vi "GEOM_SortROILevels.vi"(6 "type":enum16{"any", "normal", "rotated"}(ring), 8 "index":i32, 9 "amplifiers":T1[](array[typedef]) {"fliped" items=["none", "horizontal", "vertical"]; "type" items=["LL", "LR", "UL", "UR"]}, 10 "how":enum16{"rows (y)", "columns (x)"}(ring)) -> (1 "totpix":u32, 2 "levels":cluster{"amplifiers":i32, "coord":i32}[](array[cluster]), 4 "totdata":i32)   [LabVIEW 2016]
uses:
  GEOM_Amplifier.ctl
  GEOM_AmpType.ctl
  GEOM_ROI.ctl
  GEOM_Coords.ctl
panel:
  out "sorted amplifiers":T1[](array[typedef]) {"fliped" items=["none", "horizontal", "vertical"]; "type" items=["LL", "LR", "UL", "UR"]}
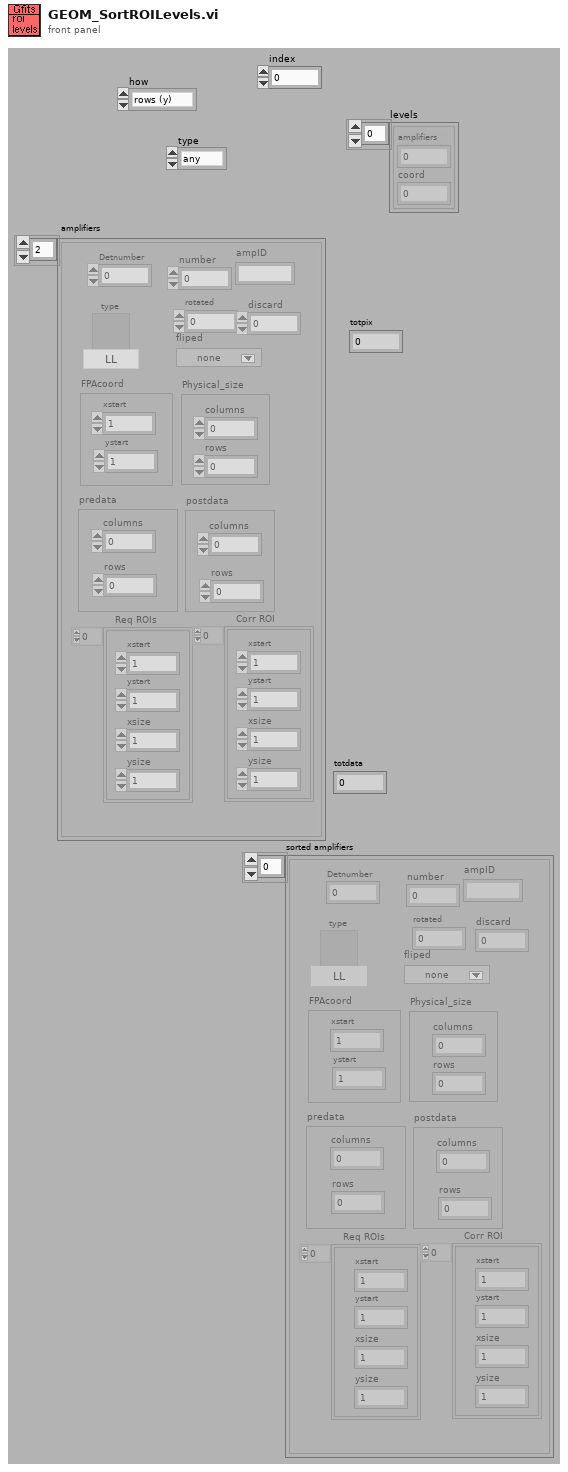
[diagram p1: front panel]
types:
  T1 = typedef "GEOM_Amplifier.ctl" = cluster{"number":i32, "type":T2, "rotated":i16, "fliped":u16, "FPAcoord":cluster{"xstart":i32, "ystart":i32}, "Physical_size":cluster{"columns":i32, "rows":i32}, "predata":cluster{"columns":i32, "rows":i32}, "postdata":cluster{"columns":i32, "rows":i32}, "Req ROIs":T3, "Corr ROI":T3, "Detnumber":i32, "ampID":string, "discard":i32}
  T2 = typedef "GEOM_AmpType.ctl" = u16
  T3 = typedef "GEOM_ROI.ctl" = T4[]
  T4 = typedef "GEOM_Coords.ctl" = cluster{"xstart":u32, "ystart":u32, "xsize":u32, "ysize":u32}
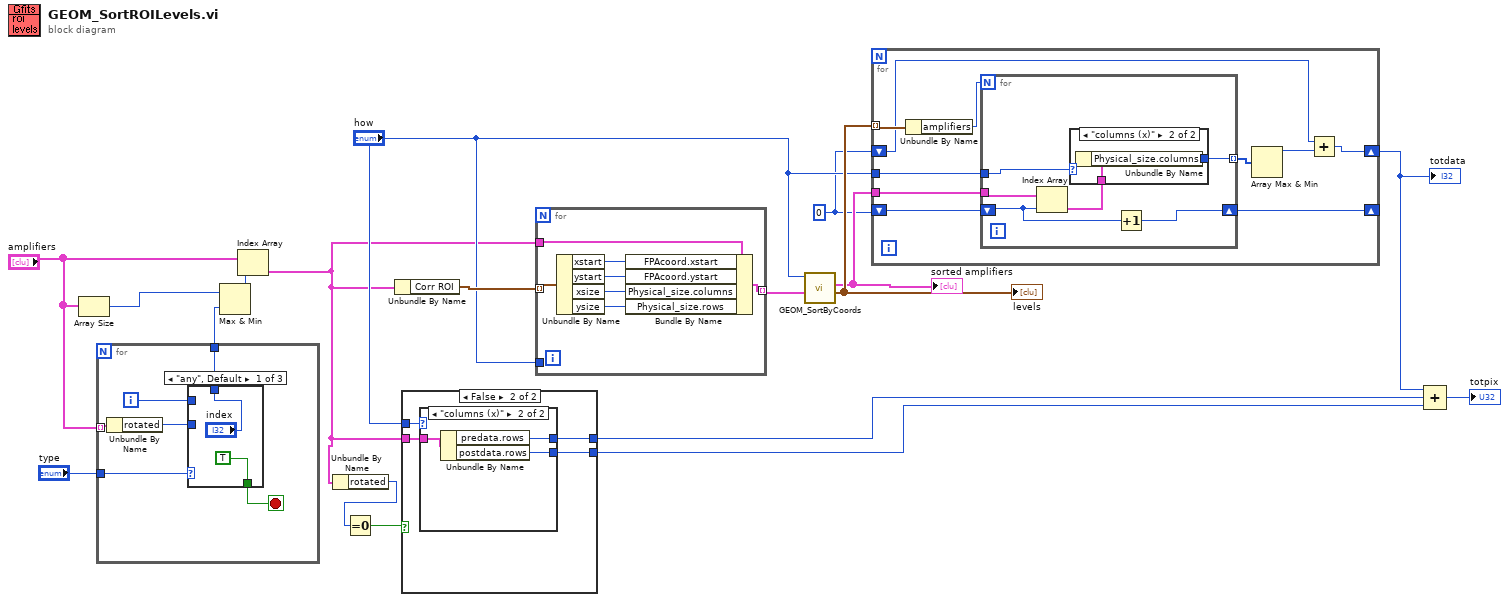
[diagram p0: block diagram]
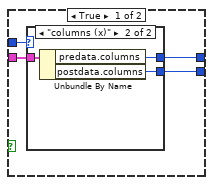
[diagram p2: hidden frame]
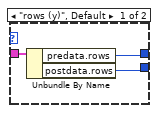
[diagram p3: hidden frame]
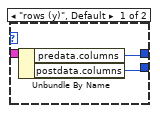
[diagram p4: hidden frame]
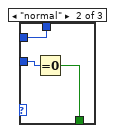
[diagram p5: hidden frame]
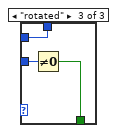
[diagram p6: hidden frame]
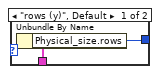
[diagram p7: hidden frame]
diagram:
  w11 = 0
  n1 = Array Size(array="amplifiers") -> (size(s)=w7:i32)
  n2 = for {
    tunnel: "amplifiers" -> [w24] mode=indexing
    tunnel: "type" -> [w23]
    tunnel: [w21] -> w5
    i -> [w20]
    stop <- w22 stop-if-true
    n3 = Unbundle By Name(w24) -> ("rotated"=w19:i16)
    n4 = case shown="\"any\", Default" w23 {
      tunnel: [TRUE w28 w31] -> w22
      tunnel: w19 -> [_ w29 w32]
      tunnel: w20 -> [_ w27 w30]
      tunnel: ["index" w27 w30] -> w21
      frame "any", Default {
      }
      frame "normal" {
        n5 = Equal To 0?(x=w29) -> (x = 0?=w28:bool)
      }
      frame "rotated" {
        n6 = Not Equal To 0?(x=w32) -> (x != 0?=w31:bool)
      }
    }
  }
  n7 = Max & Min(x=w7, y=w5) -> (min(x,y)=w6:i32)  [unwired: 1 out]
  n8 = Index Array(array="amplifiers", index=w6) -> (element=w2:T1)
  n9 = Unbundle By Name(w2) -> ("rotated"=w1:i16)
  n10 = Equal To 0?(x=w1) -> (x = 0?=w3:bool)
  n11 = Unbundle By Name(w2) -> ("Corr ROI"=w17:T3)
  n12 = case shown="False" w3 {
    tunnel: [w36 w46] -> w16
    tunnel: "how" -> [w35 w45]
    tunnel: w2 -> [w34 w44]
    tunnel: [w33 w43] -> w4
    frame True {
      n13 = case shown="\"columns (x)\"" w35 {
        tunnel: w34 -> [w39 w42]
        tunnel: [w38 w41] -> w33
        tunnel: [w37 w40] -> w36
        frame "rows (y)", Default {
          n14 = Unbundle By Name(w39) -> ("predata.rows"=w38:i32, "postdata.rows"=w37:i32)
        }
        frame "columns (x)" {
          n15 = Unbundle By Name(w42) -> ("predata.columns"=w41:i32, "postdata.columns"=w40:i32)
        }
      }
    }
    frame False {
      n16 = case shown="\"columns (x)\"" w45 {
        tunnel: w44 -> [w49 w52]
        tunnel: [w48 w51] -> w43
        tunnel: [w47 w50] -> w46
        frame "rows (y)", Default {
          n17 = Unbundle By Name(w49) -> ("predata.columns"=w48:i32, "postdata.columns"=w47:i32)
        }
        frame "columns (x)" {
          n18 = Unbundle By Name(w52) -> ("predata.rows"=w51:i32, "postdata.rows"=w50:i32)
        }
      }
    }
  }
  n19 = for {
    tunnel: w17 -> [w55] mode=indexing
    tunnel: w2 -> [w59]
    tunnel: [w56] -> w18 mode=indexing
    tunnel: "how" -> [_]
    n20 = Unbundle By Name(w55) -> ("xstart"=w58:u32, "ystart"=w57:u32, "xsize"=w54:u32, "ysize"=w53:u32)
    n21 = Bundle By Name(cluster=w59, "FPAcoord.xstart"=w58, "FPAcoord.ystart"=w57, "Physical_size.columns"=w54, "Physical_size.rows"=w53) -> (w56:T1)
  }
  n22 = call "GEOM_SortByCoords.vi"("amplifiers"=w18, "how"="how") -> ("levels"=w14:cluster{"amplifiers":i32, "coord":i32}[], "sorted amplifiers"=w13:T1[])  [unwired: 8 out]
  "levels" <- w14
  "sorted amplifiers" <- w13
  n23 = for {
    tunnel: w14 -> [w69] mode=indexing
    tunnel: w13 -> [w67]
    shift-right: [w65] -> _
    shift-left: w11 -> [w66]
    tunnel: "how" -> [w64]
    shift-right: [w60] -> w10
    shift-left: w11 -> [w61]
    n24 = Unbundle By Name(w69) -> ("amplifiers"=w68:i32)
    n25 = for {
      N: w68 -> [_]
      tunnel: w67 -> [w75]
      shift-right: [w73] -> w65
      shift-left: w66 -> [w74]
      tunnel: w64 -> [w72]
      tunnel: [w70] -> w63 mode=indexing
      n26 = Index Array(array=w75, index=w74) -> (element=w71:T1)
      n27 = case shown="\"columns (x)\"" w72 {
        tunnel: [w77 w79] -> w70
        tunnel: w71 -> [w76 w78]
        frame "rows (y)", Default {
          n28 = Unbundle By Name(w76) -> ("Physical_size.rows"=w77:i32)
        }
        frame "columns (x)" {
          n29 = Unbundle By Name(w78) -> ("Physical_size.columns"=w79:i32)
        }
      }
      n30 = Increment(x=w74) -> (x+1=w73:i32)
    }
    n31 = Array Max & Min(array=w63) -> (max value=w62:i32)  [unwired: 3 out]
    n32 = Add(x=w61, y=w62) -> (x+y=w60:i32)
  }
  "totdata" <- w10
  n33 = Compound Arithmetic op=ADD(w10, w4, w16) -> (→"totpix":i32)
